vi "setGate.vi"(2 "error in (no error)":errorcluster, 3 "Numeric":dbl, 4 "BK1823ACounter.lvclass":refnum<class "BK1823ACounter.lvclass">) -> (0 "error out":errorcluster, 1 "BK1823ACounter.lvclass 2":refnum<class "BK1823ACounter.lvclass">)   [LabVIEW 2009, in "Hardware.lvlib" / "frequencyCounters.lvlib" / "BK1823ACounter.lvclass"]
uses:
  BK1823ACounter.lvclass
  BK1823ACounter.lvclass/BK1823ACounter.ctl
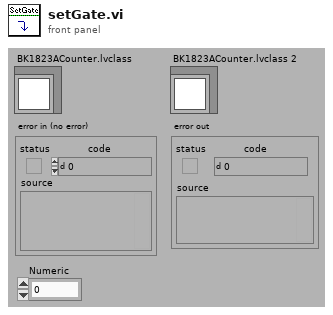
[diagram p1: front panel]
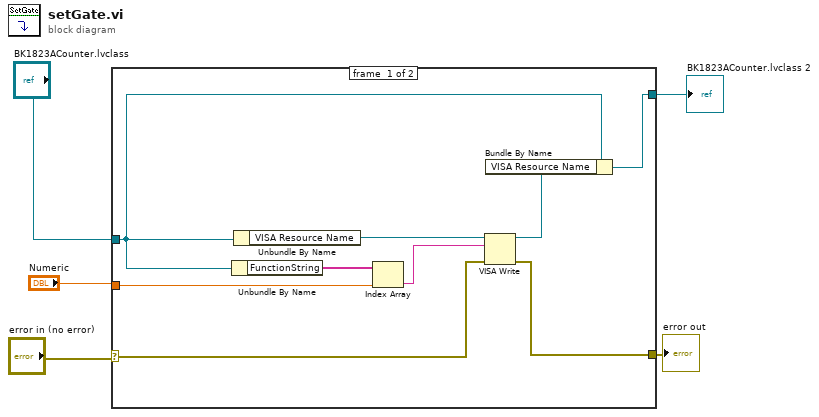
[diagram p0: block diagram]
diagram:
  n1 = case shown="No Error" "error in (no error)" {
    selector: "error in (no error)" -> [w11 w16]
    tunnel: "BK1823ACounter.lvclass" -> [w8 w15]
    tunnel: [w6 w15] -> w2
    tunnel: [w10 w16] -> w5
    tunnel: "Numeric" -> [w9 _]
    frame #0 {
      n2 = Unbundle By Name(w8) -> ("FunctionString"=w14:string[])
      n3 = Unbundle By Name(w8) -> ("VISA Resource Name"=w12:refnum<visa-resource-name>)
      n4 = Index Array(array=w14, index=w9) -> (element=w13:string)
      n5 = VISA Write(VISA resource name=w12, write buffer=w13, error in (no error)=w11) -> (VISA resource name out=w7:refnum<visa-resource-name>, error out=w10:errorcluster)  [unwired: 1 out]
      n6 = Bundle By Name(cluster=w8, "VISA Resource Name"=w7) -> (w6:refnum<class "BK1823ACounter.lvclass">)
    }
    frame #1 {
    }
  }
  "error out" <- w5
  "BK1823ACounter.lvclass 2" <- w2
